vi "-Parse_Query.vi"(8 "error in (no error)":errorcluster, 10 "Query In":string, 11 "Postgres Connector In":refnum<class "Postgres Connector.lvclass">) -> (0 "error out":errorcluster, 3 "Postgres Connector Out":refnum<class "Postgres Connector.lvclass">)   [LabVIEW 2019, in "PG_LIB.lvlib" / "Postgres Connector.lvclass"]
doc: "This VI build the query with the prefix and suffix"
uses:
  Postgres Connector.lvclass
  Postgres Connector.lvclass/Postgres Connector.ctl
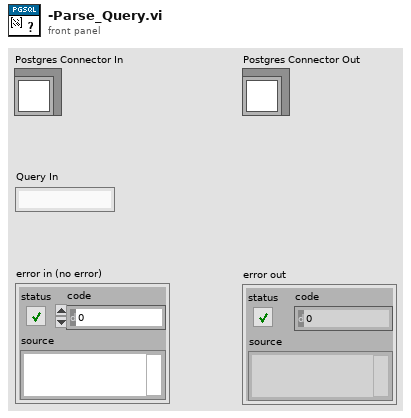
[diagram p1: front panel]
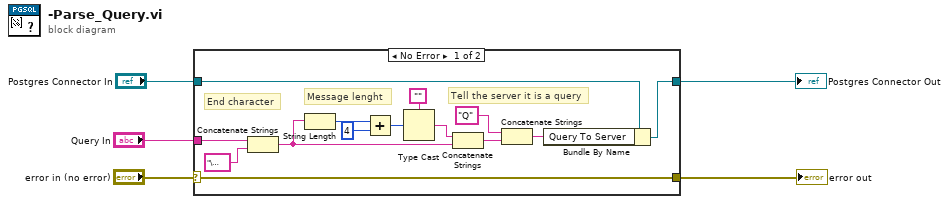
[diagram p0: block diagram]
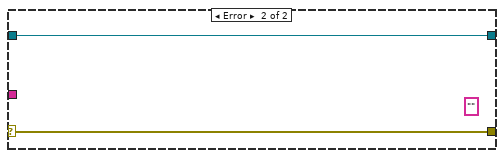
[diagram p2: hidden frame]
diagram:
  n1 = case shown="No Error" "error in (no error)" {
    selector: "error in (no error)" -> [w9 w21]
    tunnel: [w9 w21] -> w4
    tunnel: "Query In" -> [w12 _]
    tunnel: "Postgres Connector In" -> [w8 w20]
    tunnel: [w7 w20] -> w1
    frame No Error {
      # "Message lenght"
      # "Tell the server it is a query"
      # "End character"
      n2 = Concatenate Strings(w12, "\u0000") -> (w10:string)
      n3 = String Length(string=w10) -> (length=w17:i32)
      n4 = Add(x=w17, y=4) -> (x+y=w18:i32)
      n5 = Type Cast(type="", x=w18) -> (*(type *) &x=w16:string)
      n6 = Concatenate Strings(w16, w10) -> (w13:string)
      n7 = Concatenate Strings("Q", w13) -> (w6:string)
      n8 = Bundle By Name(cluster=w8, "Query To Server"=w6) -> (w7:refnum<class "Postgres Connector.lvclass">)
    }
    frame Error {
      (unwired) ""
    }
  }
  "error out" <- w4
  "Postgres Connector Out" <- w1
